vi "Create.vi"(8 "error in":errorcluster, 10 "Sub Index":u8) -> (0 "error out":errorcluster, 3 "Sub Obj out":refnum<class "Sub Object.lvclass">)   [LabVIEW 2020, in "CANopen.lvlib" / "Sub Object.lvclass"]
uses:
  Sub Object.lvclass
  Sub Object.lvclass/Sub Object.ctl
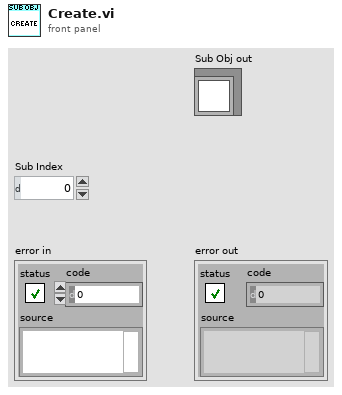
[diagram p1: front panel]
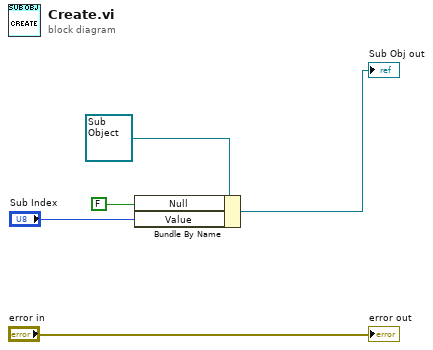
[diagram p0: block diagram]
diagram:
  n1 = Bundle By Name(cluster=refnum<class "Sub Object.lvclass"> refnum ("Object Entry"), "Null"=FALSE ("Index.Null"), "Value"="Sub Index") -> (→"Sub Obj out":refnum<class "Sub Object.lvclass">)
  "error out" <- "error in"
